vi "updata-graph-scaleSD.vi"(11 "IntensityGraph in":refnum<vi>) -> ()   [LabVIEW 2015]
uses:
  globalVarSD.vi
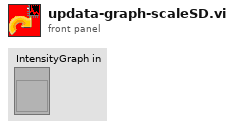
[diagram p1: front panel]
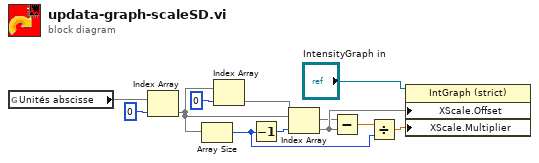
[diagram p0: block diagram]
diagram:
  n1 = global read "globalVarSD.vi" "Unités abscisse"() -> (w4)
  n2 = Index Array(array=w4, index=0 ("index (row)")) -> (element=w6)
  n3 = Array Size(array=w6) -> (size(s)=w10:i32)
  n4 = Index Array(array=w6, index=0) -> (element=w7)
  n5 = Decrement(x=w10) -> (x-1=w1:i32)
  n6 = Index Array(array=w6, index=w1) -> (element=w8)
  n7 = Subtract(x=w7, y=w8) -> (x-y=w9:dbl)
  n8 = Divide(x=w9, y=w10) -> (x/y=w11:dbl)
  n9 = property on="Property Node" class="IntGraph (strict)"(reference="IntensityGraph in", "XScale.Offset"=w8, "XScale.Multiplier"=w11) -> ()  [unwired: 1 in, 2 out]
